vi "RandomNumberGenerator_BTS.vi"(1 "Scale":dbl=25.0, 2 "Loop Count":i32=10) -> (0 "Array":dbl[](array[numeric]))   [LabVIEW 2014]
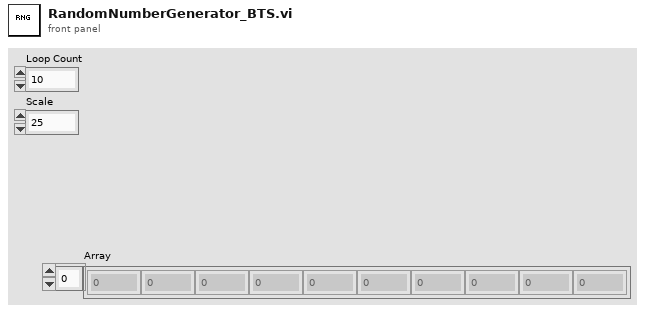
[diagram p1: front panel]
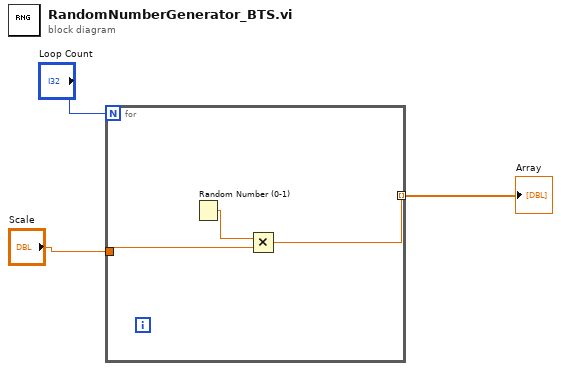
[diagram p0: block diagram]
diagram:
  n1 = for {
    N: "Loop Count" -> [_]
    tunnel: [w5] -> w2 mode=indexing
    tunnel: "Scale" -> [w4]
    n2 = Random Number (0-1)() -> (number: 0 to 1=w6:dbl)
    n3 = Multiply(x=w6, y=w4) -> (x*y=w5:dbl)
  }
  "Array" <- w2
